vi "Multiplier Channel Watcher.vi"(0 "Block Memory":refnum<k21>="Multiplier 1 Block Memory Out : [8b Identifier; 6b args; 18b fxp output]", 1 "Watched Channel":u8, 2 "Count to match":u8, 3 "Writing Index Start":u32, 4 "Timeout":i32=120) -> (5 "Writing Index End":u32, 6 "Timed out":bool, 7 "Multiplication Result":fxp<+/-,18,1> format="%.18g")   [LabVIEW 2009]
uses:
  Motor Control Global.vi
  <vilib>/Platform/TimedLoop/XDataNode/XDataNode.xnode
  <vilib>/Platform/TimedLoop/XDataNode/loadlvalarms.vi
  <vilib>/Platform/TimedLoop/XDataNode/timing_clust.ctl
  <vilib>/Platform/TimedLoop/XDataNode/nitl_modes.ctl
  <vilib>/Platform/TimedLoop/XDataNode/wakeup.ctl
  <vilib>/rvi/DataTransferAndStorage/Container/XNode/niFpgaContainer.xnode
  <vilib>/rvi/DataTransferAndStorage/Container/Common/niFpgaContainerExecOnDevCompGetState.vi
  <vilib>/rvi/DataTransferAndStorage/Container/Common/niFpgaContainerMetaDataKey.ctl
  <vilib>/rvi/Memory/Memory_Emulation/nirvimemoryEmulationManagerCache_GetValue.vi
  <vilib>/rvi/Memory/Memory_Emulation/nirvimemoryEmulationManagerCache_InsertValue.vi
  <vilib>/rvi/FIFO/Fifo_Resource/nirvififoUniquifyingName.vi
  <vilib>/Utility/error.llb/Clear Errors.vi
  <vilib>/rvi/Memory/Memory_Emulation/nirvimemoryEmulationManagerCache_SetValue.vi
  <vilib>/Platform/TimedLoop/XDataNode/XDNodeRunTimeDep.lvlib
panel:
  out "Writing Index After the best one":u32
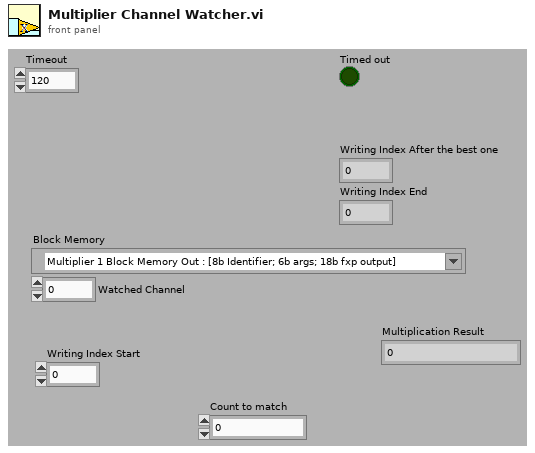
[diagram p1: front panel]
types:
  T1 = typedef "niFpgaContainerMetaDataKey.ctl" = enum16{"FPGA FIFO", "FPGA Memory", "FPGA Register"}
  T2 = typedef "XDNodeRunTimeDep.lvlib/timing_clust.ctl" = cluster{"Expected End [f-1]":u64, "Actual End [f-1]":u64, "Finished Late? [f-1]":bool, "Expected End [i-1]":u64, "Actual End [i-1]":u64, "Finished Late? [i-1]":bool, "Expected Start [i]":u64, "Actual Start [i]":u64, "Expected Start [f]":u64, "Actual Start [f]":u64, "Source Name":string, "Structure Name":string, "Period":i64, "Deadline":i64, "Offset":i64, "Start":i64, "Priority":i32, "Timeout":i32, "Mode":T3, "Wakeup Reason":T4, "Error":errorcluster, "Source Type":string, "Secondary Source Type":string, "Global End Time":u64, "Global Start Time":u64, "Frame Duration":u64, "Iteration Duration":u64, "Assigned CPU":i32, "I/O Scan Engine Mode":u32}
  T3 = typedef "XDNodeRunTimeDep.lvlib/nitl_modes.ctl" = enum32{"No Change", "Process missed periods, maintain original phase", "Discard missed periods, maintain original phase", "Process missed periods, ignore original phase", "Discard missed periods, ignore original phase"}
  T4 = typedef "XDNodeRunTimeDep.lvlib/wakeup.ctl" = enum32{"Normal", "Aborted", "Asynchronous wakeup", "Timing source error", "Timed loop error", "Timeout"}
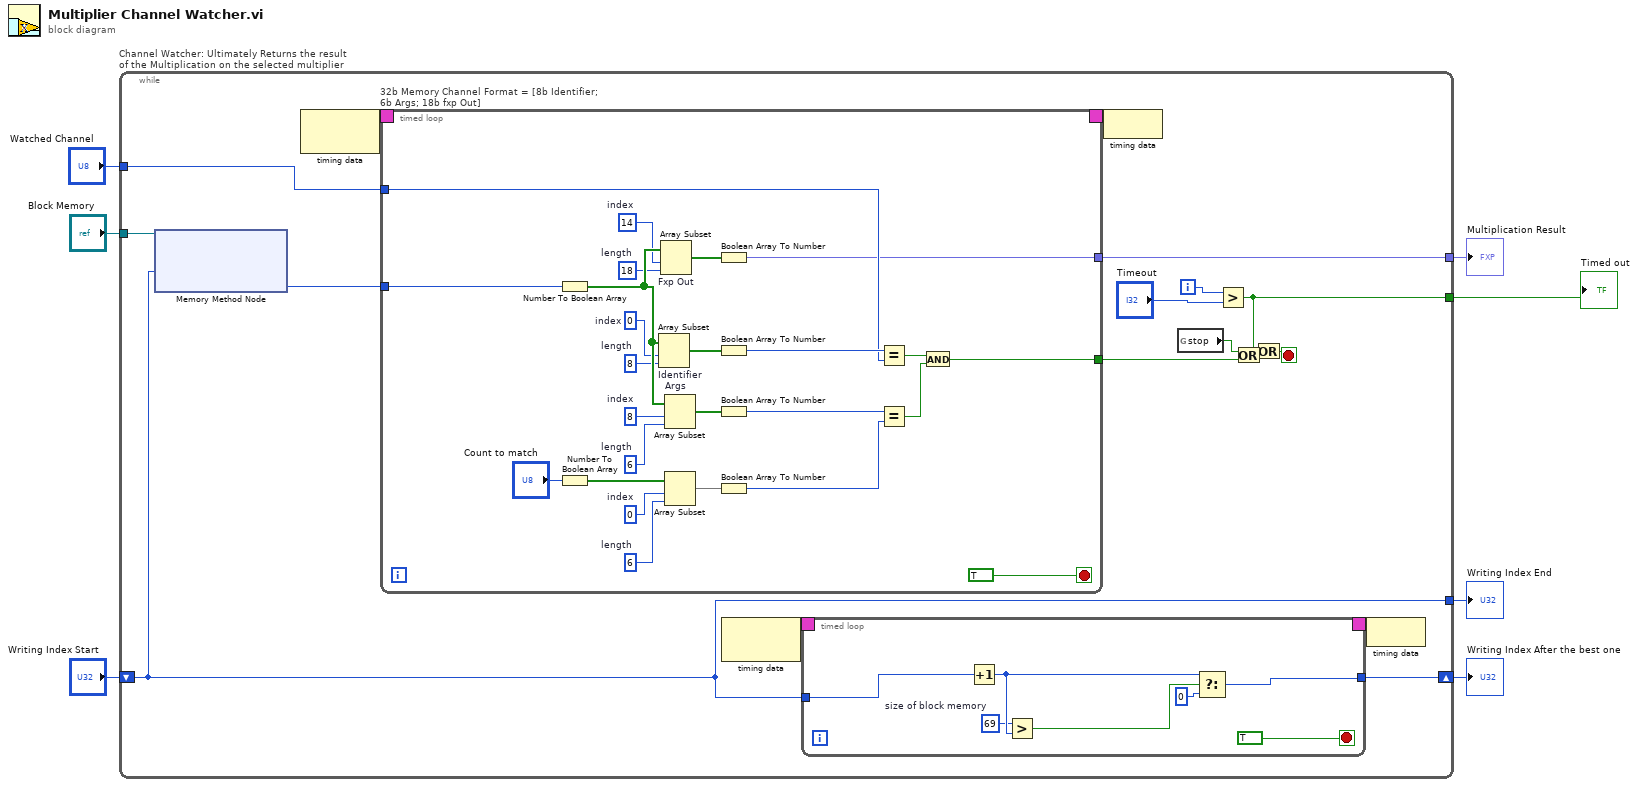
[diagram p0: block diagram]
diagram:
  n1 = while "Channel Watcher: Ultimately Returns the result of the Multiplication on the selected multiplier" {
    shift-right: [w15] -> w3
    shift-left: "Writing Index Start" -> [w12]
    tunnel: "Watched Channel" -> [w20]
    tunnel: "Block Memory" -> [w19]
    tunnel: [w18] -> w4
    tunnel: [w12] -> w2
    tunnel: [w8] -> w1
    i -> [w10]
    stop <- w9 stop-if-true
    n2 = xnode ("Memory Method Node")("Address"=w12, "Memory In"=w19) -> ("Data"=w24:u32)  [unwired: 1 out]
    n3 = node-c288() -> (w23:T2)  [unwired: 1 in]
    n4 = timed-loop "32b Memory Channel Format = [8b Identifier; 6b Args; 18b fxp Out]" {
      timing: w23 -> [_]
      timing-out: [_] -> w22
      tunnel: w24 -> [w49]
      tunnel: w20 -> [w48]
      tunnel: [w47] -> w18
      tunnel: [w46] -> w16
      stop <- TRUE stop-if-true
      w39 = 6  # length
      w40 = 0  # index
      w54 = 8  # length
      w55 = 6  # length
      w56 = 18  # length
      w57 = 14  # index
      w58 = 8  # index
      w59 = 0  # index
      n5 = Number To Boolean Array(number=w49) -> (Boolean array=w60:bool[])
      n6 = Number To Boolean Array(number="Count to match") -> (Boolean array=w42:bool[])
      n7 = Array Subset "Identifier"(array=w60, index=w59, length=w54) -> (w53:bool[])
      n8 = Array Subset "Fxp Out"(array=w60, index=w57, length=w56) -> (w52:bool[])
      n9 = Array Subset "Args"(array=w60, index=w58, length=w55) -> (w44:bool[])
      n10 = Array Subset(array=w42, index=w40, length=w39) -> (w41:bool[])
      n11 = Boolean Array To Number(Boolean array=w52) -> (number=w47:fxp<+/-,18,1>)
      n12 = Boolean Array To Number(Boolean array=w53) -> (number=w51:u8)
      n13 = Boolean Array To Number(Boolean array=w44) -> (number=w38:u8)
      n14 = Boolean Array To Number(Boolean array=w41) -> (number=w37:u8)
      n15 = Equal?(x=w51, y=w48) -> (x = y?=w50:bool)
      n16 = Equal?(x=w38, y=w37) -> (x = y?=w36:bool)
      n17 = And ("We have what we want")(x=w50, y=w36) -> (x .and. y?=w46:bool)
    }
    n18 = node-c288() -> (w14:T2)  [unwired: 1 in]
    n19 = timed-loop {
      timing: w14 -> [_]
      timing-out: [_] -> w13
      tunnel: w12 -> [w27]
      tunnel: [w26] -> w15
      stop <- TRUE stop-if-true
      w29 = u32 69  # size of block memory
      n20 = Increment(x=w27) -> (x+1=w30:u32)
      n21 = Greater?(x=w29, y=w30) -> (0:w28:bool)
      n22 = Select(t=w30, s=w28, f=u32 0) -> (s? t:f=w26:u32)
    }
    n23 = node-c288(w22) -> ()
    n24 = global read "Motor Control Global.vi" "stop"() -> (w21:bool)
    n25 = Greater?(x=w10, y="Timeout") -> (0:w8:bool)
    n26 = Or(x=w21, y=w16) -> (x .or. y?=w17:bool)
    n27 = Or(x=w8, y=w17) -> (x .or. y?=w9:bool)
    n28 = node-c288(w13) -> ()
  }
  "Multiplication Result" <- w4
  "Writing Index After the best one" <- w3
  "Writing Index End" <- w2
  "Timed out" <- w1
